vi "PrecentFull.vi"(3 "Image In":T1 {"Dialogs" format="%.0b"}) -> (0 "% solid":dbl, 1 "Image Out":T1 {"Dialogs" format="%.0b"})   [LabVIEW 2024]
doc: "This VI takes any image in as an input. It return a value equal to the percentage of pixels in the image that are 1 (binary images) or 255 (8 bit Grey or RGB images)."
uses:
  <userlib>/ImageProcessing/QTLIB_2595_LV86/QT_Image.ctl
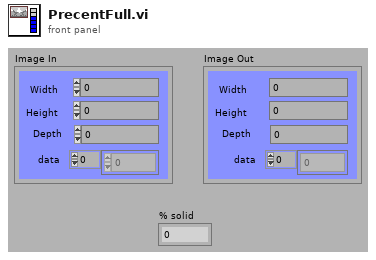
[diagram p1: front panel]
types:
  T1 = typedef "QT_Image.ctl" = cluster{"Width":i32, "Height":i32, "Depth":i32, "data":u8[], "Compressed data":u8[], "Color table":u32[], "Duration":i32, "Options":i32, "Timestamp":i32, "ID":i32, "Reserved":i32, "Dialogs":u32}
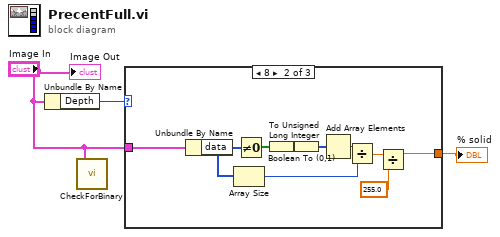
[diagram p0: block diagram]
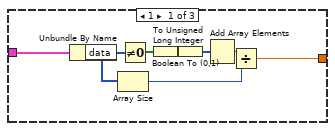
[diagram p2: hidden frame]
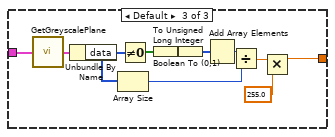
[diagram p3: hidden frame]
diagram:
  n1 = Unbundle By Name("Image In") -> ("Depth"=w2:i32)
  n2 = call <userlib>:"CheckForBinary.vi"("Image in"="Image In") -> ()  [unwired: 2 in, 1 out]
  n3 = case shown="8" w2 {
    tunnel: "Image In" -> [w11 w21 w32]
    tunnel: [w5 w13 w24] -> w3
    frame 1 {
      n4 = Unbundle By Name(w11) -> ("data"=w7:u8[])
      n5 = Array Size(array=w7) -> (size(s)=w6:i32)
      n6 = Not Equal To 0?(x=w7) -> (x != 0?=w10:bool[])
      n7 = Boolean To (0,1)(Boolean=w10) -> (0, 1=w9:i16[])
      n8 = To Unsigned Long Integer(number=w9) -> (unsigned 32bit integer=w4:u32[])
      n9 = Add Array Elements(numeric array=w4) -> (sum=w8:u32)
      n10 = Divide(x=w8, y=w6) -> (x/y=w5:dbl)
    }
    frame 8 {
      n11 = Unbundle By Name(w21) -> ("data"=w17:u8[])
      n12 = Array Size(array=w17) -> (size(s)=w16:i32)
      n13 = Not Equal To 0?(x=w17) -> (x != 0?=w20:bool[])
      n14 = Boolean To (0,1)(Boolean=w20) -> (0, 1=w19:i16[])
      n15 = To Unsigned Long Integer(number=w19) -> (unsigned 32bit integer=w15:u32[])
      n16 = Add Array Elements(numeric array=w15) -> (sum=w18:u32)
      n17 = Divide(x=w18, y=w16) -> (x/y=w14:dbl)
      n18 = Divide(x=w14, y=255.0) -> (x/y=w13:dbl)
    }
    frame Default {
      n19 = call <userlib>:"GetGreyscalePlane.vi"("Image In"=w32) -> ("Greyscale  Out"=w22:T1)
      n20 = Unbundle By Name(w22) -> ("data"=w28:u8[])
      n21 = Array Size(array=w28) -> (size(s)=w27:i32)
      n22 = Not Equal To 0?(x=w28) -> (x != 0?=w31:bool[])
      n23 = Boolean To (0,1)(Boolean=w31) -> (0, 1=w30:i16[])
      n24 = To Unsigned Long Integer(number=w30) -> (unsigned 32bit integer=w26:u32[])
      n25 = Add Array Elements(numeric array=w26) -> (sum=w29:u32)
      n26 = Divide(x=w29, y=w27) -> (x/y=w25:dbl)
      n27 = Multiply(x=w25, y=255.0) -> (x*y=w24:dbl)
    }
  }
  "% solid" <- w3
  "Image Out" <- "Image In"
